vi "Check Thermocouple.vi"(8 "error in (no error)":errorcluster, 11 "Freezer in":refnum<class "Freezer.lvclass">) -> (0 "error out":errorcluster, 1 "In Range?":bool, 2 "data out":dbl, 3 "Freezer out":refnum<class "Freezer.lvclass">)   [LabVIEW 2015, in "cRIO-Carbondioxide.lvlib" / "CO2-Actor.lvlib" / "Freezer.lvclass"]
uses:
  Freezer.lvclass
  Freezer.lvclass/Freezer.ctl
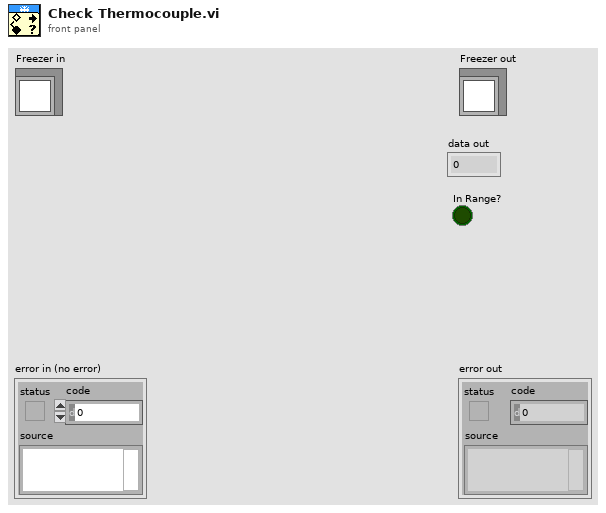
[diagram p1: front panel]
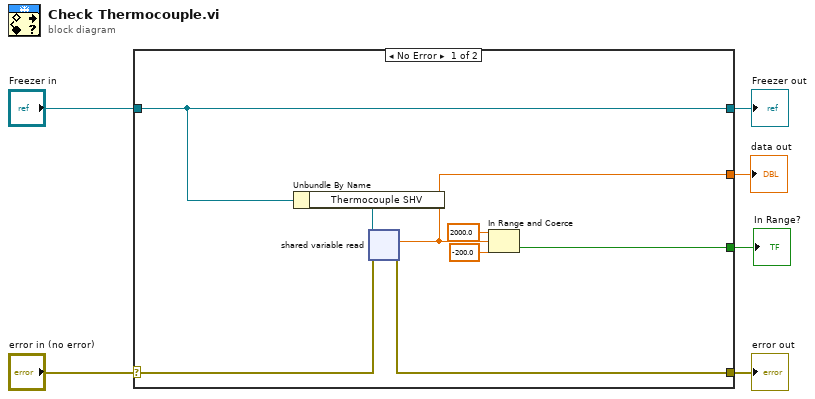
[diagram p0: block diagram]
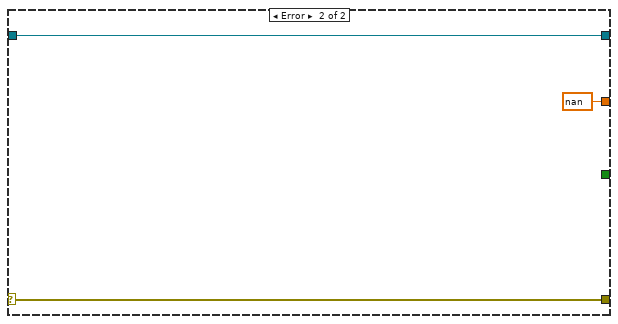
[diagram p2: hidden frame]
diagram:
  n1 = case shown="No Error" "error in (no error)" {
    selector: "error in (no error)" -> [w10 w17]
    tunnel: [w9 w17] -> w5
    tunnel: [w11 w16] -> w3
    tunnel: "Freezer in" -> [w11 w16]
    tunnel: [w8 _] -> w2
    tunnel: [w7 nan ("Syringe TC")] -> w1
    frame No Error {
      n2 = Unbundle By Name(w11) -> ("Thermocouple SHV"=w14:refnum<k21>)
      n3 = shared-variable-read(w14, w10) -> (w9:errorcluster, w7:dbl)  [unwired: 2 out]
      n4 = In Range and Coerce(upper limit=2000.0, x=w7, lower limit=-200.0) -> (In Range?=w8:bool)  [unwired: 1 out]
    }
    frame Error {
    }
  }
  "error out" <- w5
  "Freezer out" <- w3
  "In Range?" <- w2
  "data out" <- w1
